vi "Get Fixed Wheel Information.vi"(8 "error in (no error)":errorcluster, 11 "wheel in":refnum<class "NI_Robotics_Wheel.lvclass">) -> (0 "error out":errorcluster, 1 "wheel name":string, 2 "wheel parameters":T1={"wheel radius"=1.0, "gear ratio"=1.0, "forward rotation direction"=0} {"forward rotation direction" items=["Clockwise", "Counterclockwise"]}, 3 "wheel out":refnum<class "NI_Robotics_Wheel.lvclass">, 4 "motor communication":refnum<class "NI_Robotics_Motor Communication.lvclass">)   [LabVIEW 2017, in "NI_Robotics_Wheel.lvclass"]
doc: "Returns information, such as <B>wheel radius</B> and <B>gear ratio</B>, for the wheel you specify. You must manually select the polymorphic instance to use."
uses:
  <vilib>/robotics/Steering/Wheel/NI_Robotics_Wheel.lvclass
  <vilib>/robotics/Steering/Wheel/Wheel Parameters.ctl
  <vilib>/robotics/Steering/Wheel/Rotation Direction.ctl
  <vilib>/robotics/Actuation/Motor Communication/NI_Robotics_Motor Communication.lvclass
  <vilib>/robotics/Steering/Fixed Wheel/NI_Robotics_Fixed Wheel.lvclass
  c:/Program Files (x86)/National Instruments/LabVIEW 2017/vi.lib/robotics/Steering/Wheel/NI_Robotics_Wheel.lvclass
  <vilib>/robotics/Steering/Wheel/NI_Robotics_Wheel.lvclass/NI_Robotics_Wheel.ctl
  <vilib>/robotics/Steering/Wheel/Get Motor Communication.vi
  <vilib>/robotics/Steering/Wheel/Get Wheel Parameters.vi
  <vilib>/robotics/Utilities/Generate Error.vi
  <vilib>/robotics/Utilities/Clear Specific Error.vi
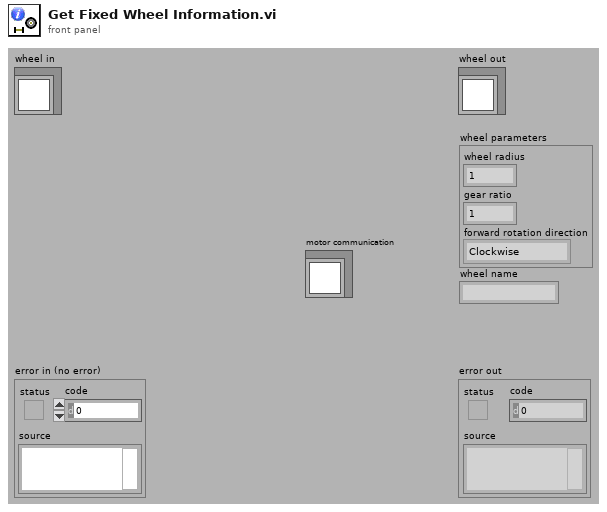
[diagram p1: front panel]
types:
  T1 = typedef "NI_Robotics_Wheel.lvclass/Wheel Parameters.ctl" = cluster{"wheel radius":dbl, "gear ratio":dbl, "forward rotation direction":T2}
  T2 = typedef "NI_Robotics_Wheel.lvclass/Rotation Direction.ctl" = u16
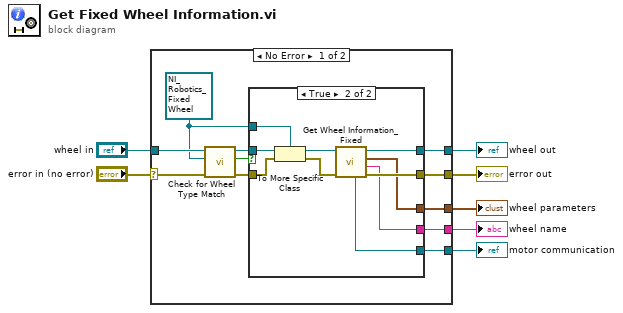
[diagram p0: block diagram]
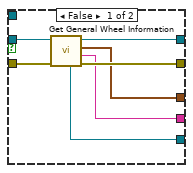
[diagram p2: hidden frame]
diagram:
  n1 = case shown="No Error" "error in (no error)" {
    selector: "error in (no error)" -> [w10 w37]
    tunnel: [w17 w37] -> w6
    tunnel: [w18 w36] -> w4
    tunnel: "wheel in" -> [w13 w36]
    tunnel: [w16 _] -> w3
    tunnel: [w15 _] -> w2
    tunnel: [w14 _] -> w1
    frame No Error {
      w8 = refnum<class "NI_Robotics_Fixed Wheel.lvclass"> refnum ("fixed wheel in")
      n2 = call <vilib>:"Check for Wheel Type Match.vi"("error in (no error)"=w10, "target wheel type"=w8, "wheel in"=w13) -> ("error out"=w11:errorcluster, "match?"=w12:bool, "wheel out"=w9:refnum<class "NI_Robotics_Wheel.lvclass">)  [unwired: 6 in]
      n3 = case shown="True" w12 {
        tunnel: w9 -> [w25 w28]
        tunnel: [w23 w35] -> w18
        tunnel: [w22 w34] -> w17
        tunnel: [w21 w33] -> w16
        tunnel: [w20 w32] -> w15
        tunnel: [w19 w31] -> w14
        tunnel: w11 -> [w24 w30]
        tunnel: w8 -> [_ w26]
        frame False {
          n4 = call <vilib>:"Get General Wheel Information.vi"("error in (no error)"=w24, "wheel in"=w25) -> ("error out"=w22:errorcluster, "wheel name"=w20:string, "wheel parameters"=w21:T1, "wheel out"=w23:refnum<class "NI_Robotics_Wheel.lvclass">, "motor communication"=w19:refnum<class "NI_Robotics_Motor Communication.lvclass">)  [unwired: 5 in]
        }
        frame True {
          n5 = To More Specific Class(target class=w26, reference=w28, error in=w30) -> (specific class reference=w27:refnum<class "NI_Robotics_Fixed Wheel.lvclass">, error out=w29:errorcluster)
          n6 = call <vilib>:"Get Wheel Information_Fixed.vi"("error in (no error)"=w29, "fixed wheel in"=w27) -> ("error out"=w34:errorcluster, "wheel name"=w32:string, "wheel parameters"=w33:T1, "fixed wheel out"=w35:refnum<class "NI_Robotics_Fixed Wheel.lvclass">, "motor communication"=w31:refnum<class "NI_Robotics_Motor Communication.lvclass">)  [unwired: 5 in]
        }
      }
    }
    frame Error {
    }
  }
  "error out" <- w6
  "wheel out" <- w4
  "wheel parameters" <- w3
  "wheel name" <- w2
  "motor communication" <- w1
